vi "checkStopReading.vi"(8 "error in (no error)":errorcluster, 10 "endReading?":bool, 11 "ElectrometerController in":refnum<class "ElectrometerController.lvclass">) -> (0 "error out":errorcluster, 3 "ElectrometerController out":refnum<class "ElectrometerController.lvclass">)   [LabVIEW 2016, in "ElectrometerController.lvclass"]
uses:
  ElectrometerController.lvclass
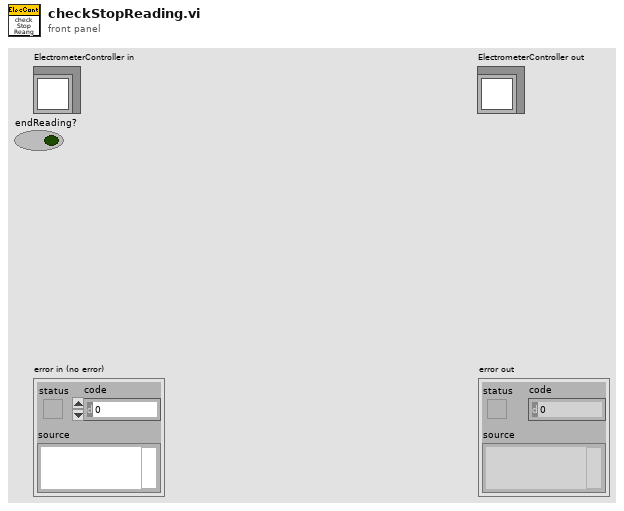
[diagram p1: front panel]
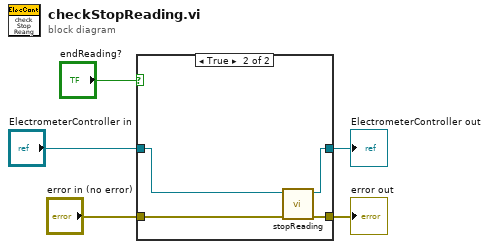
[diagram p0: block diagram]
diagram:
  n1 = case shown="True" "endReading?" {
    tunnel: "error in (no error)" -> [w6 w10]
    tunnel: [w6 w9] -> w4
    tunnel: "ElectrometerController in" -> [w7 w11]
    tunnel: [w7 w8] -> w2
    frame False {
    }
    frame True {
      n2 = call "stopReading.vi"("error in (no error)"=w10, "ElectrometerController in"=w11) -> ("error out"=w9:errorcluster, "ElectrometerController out"=w8:refnum<class "ElectrometerController.lvclass">)  [unwired: 8 in]
    }
  }
  "error out" <- w4
  "ElectrometerController out" <- w2
